vi "Winch.vi"() -> ()   [LabVIEW 2013]
uses:
  Globals/Homes.vi
  <vilib>/Rock Robotics/WPI/Joystick/WPI_JoystickGetSetRefNum.vi
  Robot Global Data.vi
  <vilib>/addons/control/pid/pid.llb/PID (DBL).vi
  <vilib>/addons/control/pid/NI_PID_pid.lvlib
panel:
  out "x-y":dbl
  out "Setpoint":dbl
  out "Motor Output":dbl
  out "Winch Voltage":dbl=2.9095941520000004
  in  "PID gains":T1={"proportional gain (Kc)"=2.75, "integral time (Ti, min)"=0.0, "derivative time (Td, min)"=0.0} {"derivative time (Td, min)" format="%.3f"; "integral time (Ti, min)" format="%.3f"; "proportional gain (Kc)" format="%.3f"}
  # "4.3"
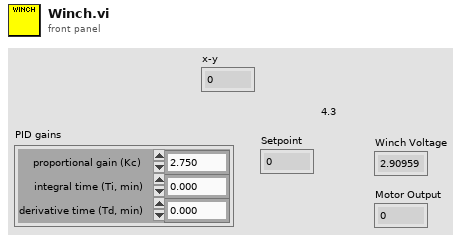
[diagram p1: front panel]
types:
  T1 = cluster{"proportional gain (Kc)":dbl, "integral time (Ti, min)":dbl, "derivative time (Td, min)":dbl}
  T2 = typedef "WPI_JoystickDevRef.ctl" = cluster{"Device":T3}
  T3 = typedef "WPI_JoystickDeviceEnum.ctl" = enum16{"USB 1", "USB 2", "USB 3", "USB 4", "Kinect 1", "Kinect 2"}
  T4 = typedef "WPI_AnalogChannelDevRef.ctl" = cluster{"DevStatus":errorcluster, "Analog Module":T5, "Analog Channel":T6}
  T5 = typedef "FPGA_TypedefAnalogModule.ctl" = enum16{"Analog Module 1", "Analog Module 2"}
  T6 = typedef "FPGA_AIChannel.ctl" = enum8{"AI 1", "AI 2", "AI 3", "AI 4", "AI 5", "AI 6", "AI 7", "AI 8", "Invalid"}
  T7 = typedef "WPI_MotorControlDeviceRef.ctl" = cluster{"DeviceStatus":errorcluster, "Type":enum16{"PWM", "CAN"}, "PWM":cluster{"Digital Module":T8, "PWM Channel":T9, "DeadBand":T10}, "CAN":cluster{"Device Number":u8, "Control Mode":T11, "Semaphore":T12, "Max Vout":dbl}, "Invert":bool, "TransformRef":T13, "InvTransformRef":T13}
  T8 = typedef "FPGA_TypedefDigitalModule.ctl" = enum16{"Digital Module 1", "Digital Module 2"}
  T9 = typedef "FPGA_DIOPWMChannel.ctl" = enum8{"PWM 1", "PWM 2", "PWM 3", "PWM 4", "PWM 5", "PWM 6", "PWM 7", "PWM 8", "PWM 9", "PWM 10", "Invalid"}
  T10 = typedef "WPI_PWMDeadband.ctl" = cluster{"Name":string, "maxPositivePwm":i32, "minPositivePwm":i32, "centerPwm":i32, "maxNegativePwm":i32, "minNegativePwm":i32, "angularRange":u16}
  T11 = typedef "WPI_CANJaguar_ControlMode.ctl" = enum8{"Percent VBus", "Current", "Speed", "Position", "Voltage"}
  T12 = typedef "Semaphore RefNum" = refnum<k1>
  T13 = typedef "WPI_PWMTransform_ConPane.ctl" = refnum<vi>
  T14 = typedef "WPI_DriverStationRobotMode2.ctl" = enum16{"Autonomous Disabled", "Autonomous Enabled", "Teleop Disabled", "Teleop Enabled", "Timeout", "Finish", "Test Disabled", "Test Enabled"}
  T15 = typedef "WPI_JoystickButtonState.ctl" = cluster{"Button 1":bool, "Button 2":bool, "Button 3":bool, "Button 4":bool, "Button 5":bool, "Button 6":bool, "Button 7":bool, "Button 8":bool, "Button 9":bool, "Button 10":bool, "Button 11":bool, "Button 12":bool}
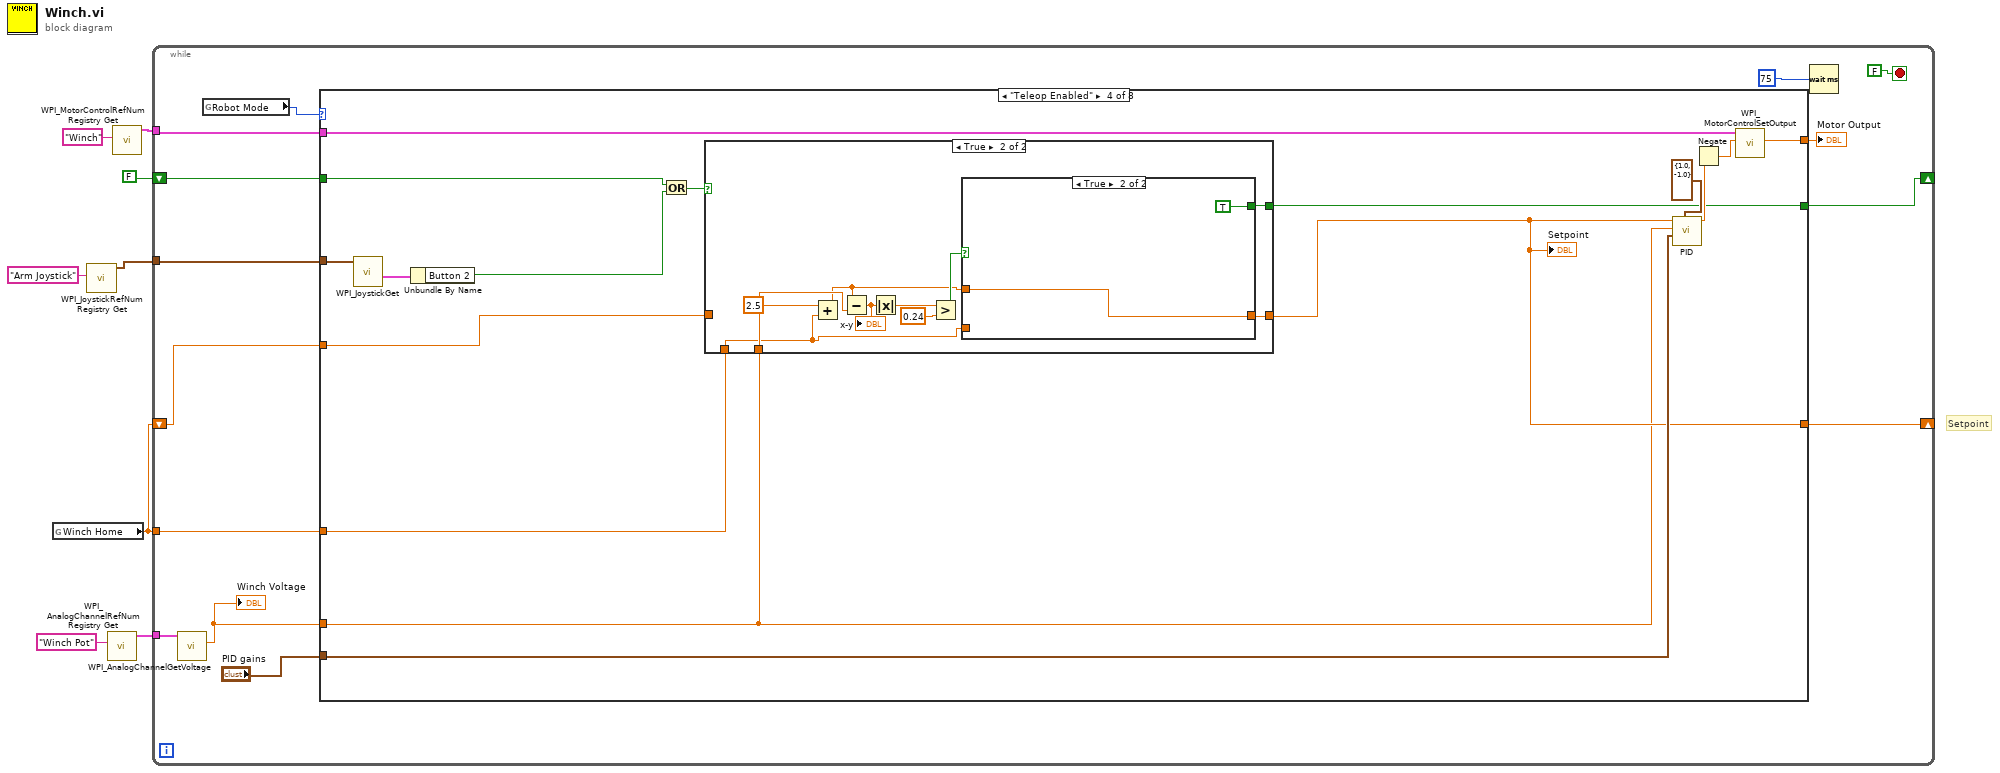
[diagram p0: block diagram]
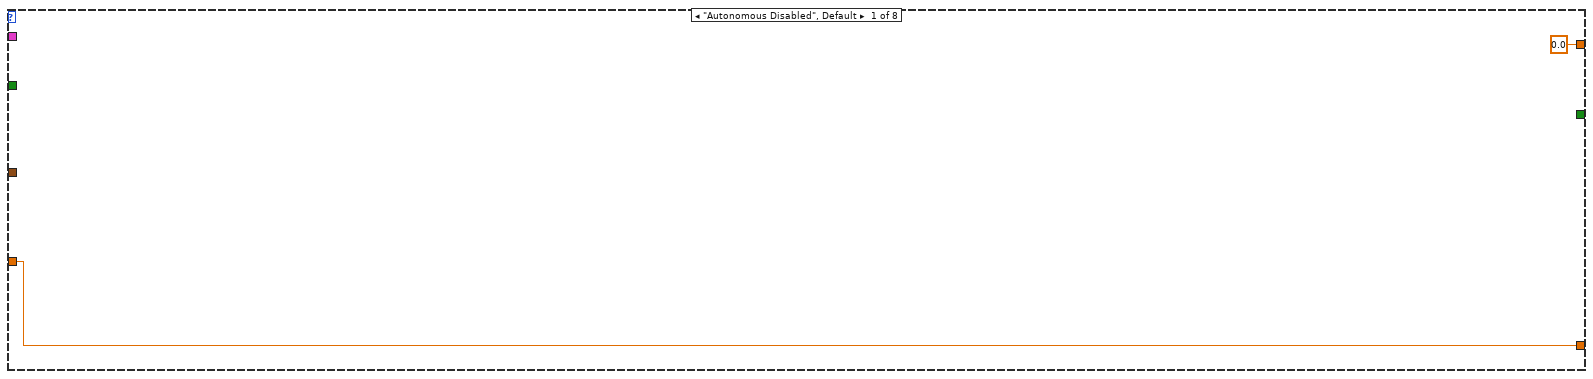
[diagram p2: hidden frame]
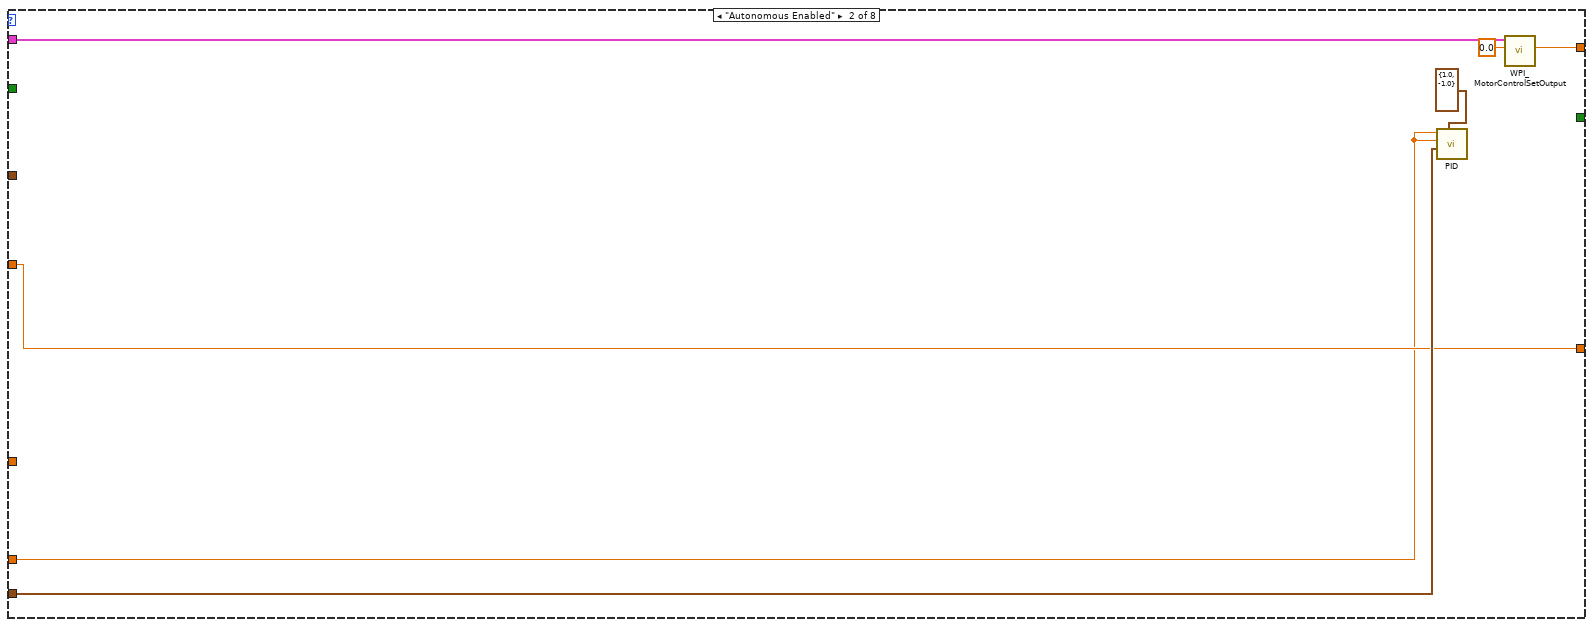
[diagram p3: hidden frame]
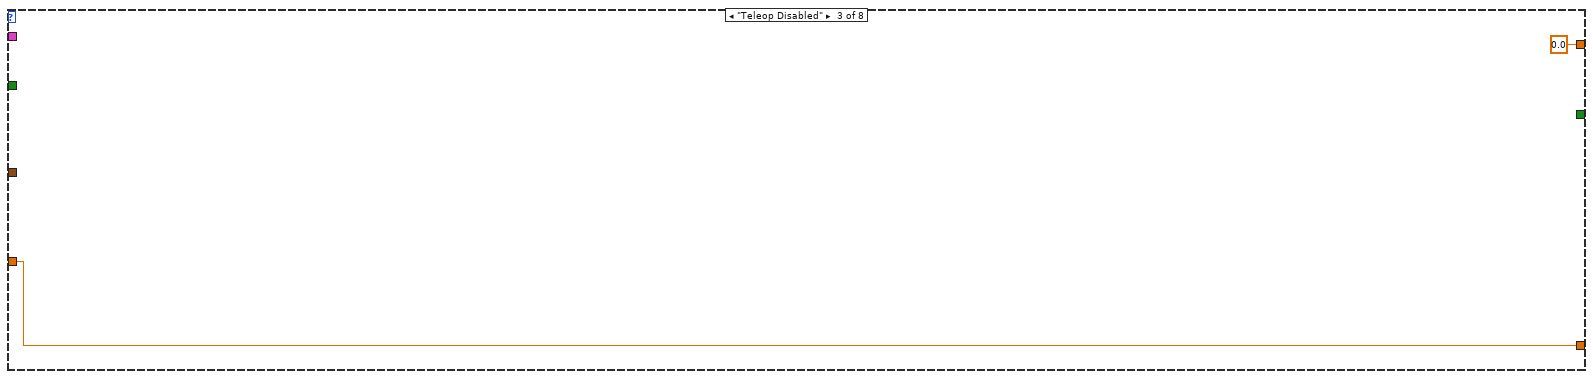
[diagram p4: hidden frame]
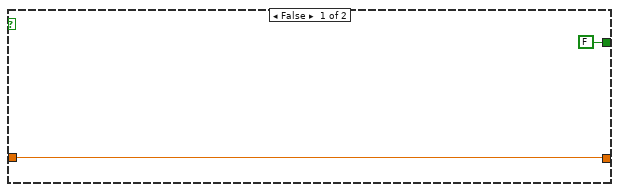
[diagram p5: hidden frame]
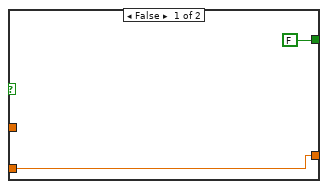
[diagram p6: hidden frame]
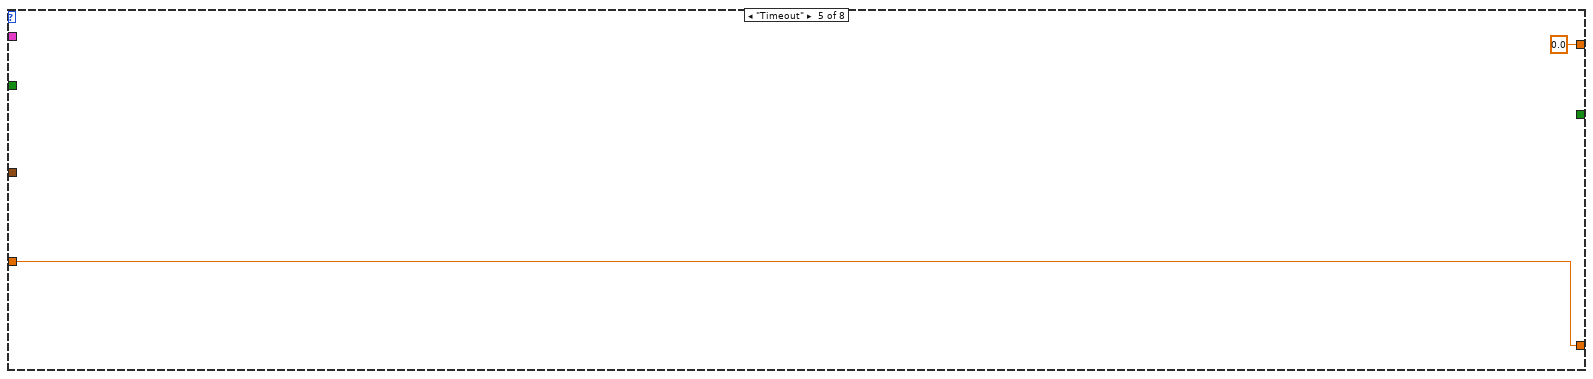
[diagram p7: hidden frame]
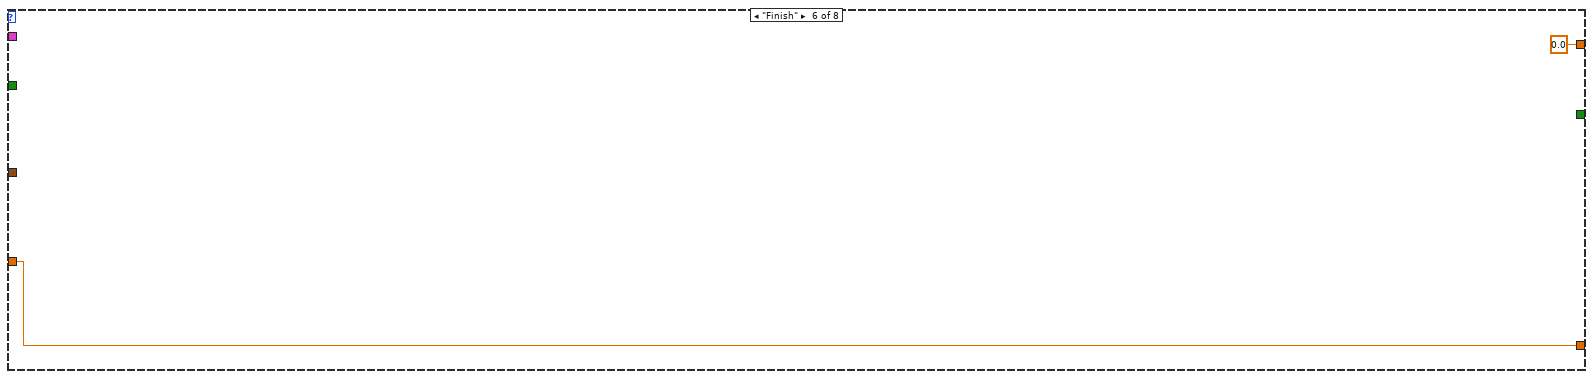
[diagram p8: hidden frame]
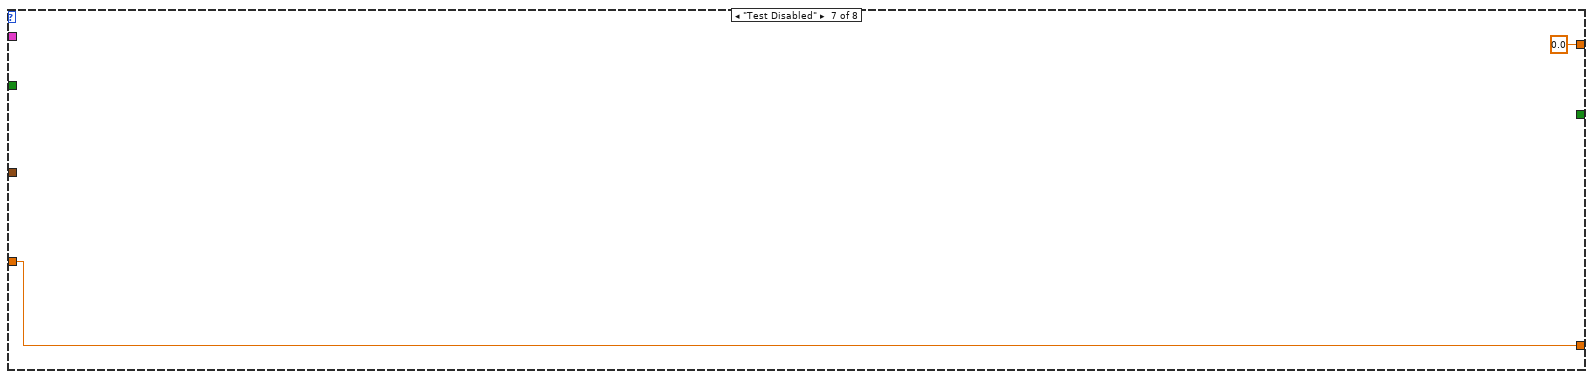
[diagram p9: hidden frame]
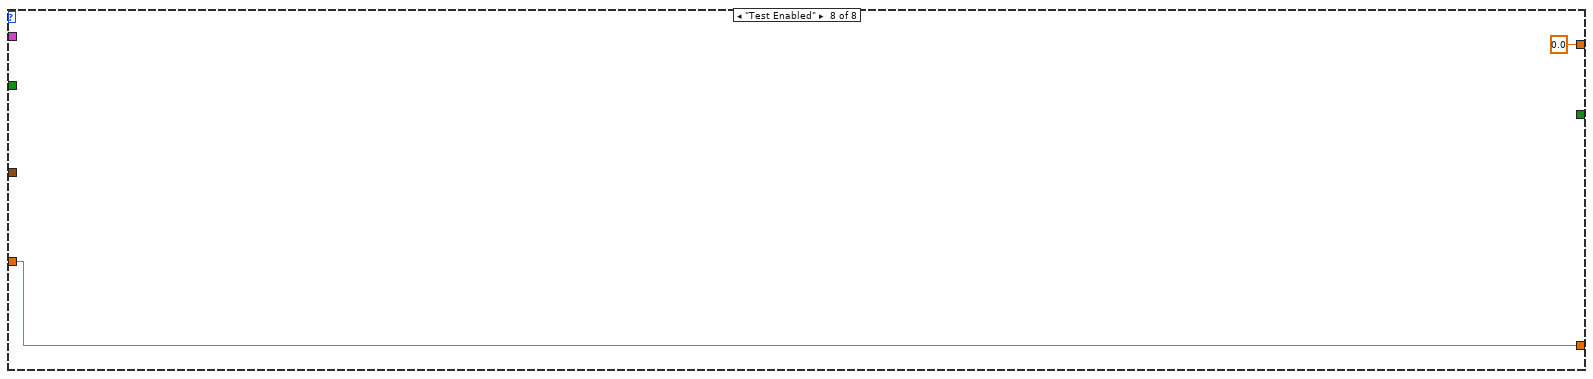
[diagram p10: hidden frame]
diagram:
  # "Setpoint"
  n1 = global read "Homes.vi" "Winch Home"() -> (w4:dbl)
  n2 = call <vilib>:"WPI_JoystickRefNum Registry Get.vi"("refnum name"="Arm Joystick") -> ("JoystickDevRef"=w2:T2)  [unwired: 9 in, 1 out]
  n3 = call <vilib>:"WPI_AnalogChannelRefNum Registry Get.vi"("refnum name"="Winch Pot") -> ("AIDeviceRef"=w8:T4)  [unwired: 9 in, 1 out]
  n4 = call <vilib>:"WPI_MotorControlRefNum Registry Get.vi"("refnum name"="Winch") -> ("MotorControlDevRef"=w5:T7)  [unwired: 9 in, 1 out]
  n5 = while {
    tunnel: w8 -> [w20]
    tunnel: w5 -> [w18]
    tunnel: w4 -> [w12]
    shift-right: [w11] -> _
    shift-left: w4 -> [w13]
    tunnel: w2 -> [w14]
    shift-right: [w9] -> _
    shift-left: FALSE ("Button 2") -> [w10]
    stop <- FALSE stop-if-true
    n6 = call <vilib>:"WPI_AnalogChannelGetVoltage.vi"("AIDeviceRef"=w20) -> ("Voltage"=w17:dbl)  [unwired: 8 in, 2 out]
    "Winch Voltage" <- w17
    n7 = global read "Robot Global Data.vi" "Robot Mode"() -> (w19:T14)
    n8 = case shown="\"Teleop Enabled\"" w19 {
      tunnel: w18 -> [_ w29 _ w48 _ _ _ _]
      tunnel: w17 -> [_ w26 _ w36 _ _ _ _]
      tunnel: "PID gains" -> [_ w30 _ w47 _ _ _ _]
      tunnel: [0.0 ("Motor Output") w28 0.0 ("Motor Output") w46 0.0 ("Motor Output") 0.0 ("Motor Output") 0.0 ("Motor Output") 0.0 ("Motor Output")] -> w15
      tunnel: w14 -> [_ _ _ w44 _ _ _ _]
      tunnel: w13 -> [w23 w27 w32 w40 w66 w68 w70 w72]
      tunnel: w12 -> [_ _ _ w42 _ _ _ _]
      tunnel: [w23 w27 w32 w41 w66 w68 w70 w72] -> w11
      tunnel: w10 -> [_ _ _ w37 _ _ _ _]
      tunnel: [_ _ _ w35 _ _ _ _] -> w9
      frame "Autonomous Disabled", Default {
      }
      frame "Autonomous Enabled" {
        n9 = call-poly <vilib>:"PID.vi"("output range"=cluster{"output high":dbl, "output low":dbl} {"output high"=1.0, "output low"=-1.0}, "PID gains"=w30, "process variable"=w26, "setpoint"=w26) -> ()  [unwired: 6 in, 2 out]
        n10 = call <vilib>:"WPI_MotorControlSetOutput.vi"("Output"=0.0, "MotorControlDevRef"=w29) -> ("Motor Output"=w28:dbl)  [unwired: 7 in, 2 out]
      }
      frame "Teleop Disabled" {
      }
      frame "Teleop Enabled" {
        n11 = call <vilib>:"WPI_JoystickGet.vi"("JoystickDevRef"=w44) -> ("Buttons"=w43:T15)  [unwired: 4 in, 2 out]
        n12 = Unbundle By Name(w43) -> ("Button 2"=w38:bool)
        n13 = Or(x=w37, y=w38) -> (x .or. y?=w39:bool)
        n14 = case shown="True" w39 {
          tunnel: w42 -> [_ w53]
          tunnel: [w51 w55] -> w41
          tunnel: w40 -> [w51 _]
          tunnel: w36 -> [_ w60]
          tunnel: [FALSE w52] -> w35
          frame False {
          }
          frame True {
            n15 = Add(x=2.5 ("Offset"), y=w53) -> (x+y=w54:dbl)
            n16 = Subtract(x=w54, y=w60) -> (x-y=w59:dbl)
            "x-y" <- w59
            n17 = Absolute Value(x=w59) -> (abs(x)=w58:dbl)
            n18 = Greater?(x=w58, y=0.24) -> (0:w56:bool)
            n19 = case shown="True" w56 {
              tunnel: [w63 w65] -> w55
              tunnel: w54 -> [_ w65]
              tunnel: w53 -> [w63 _]
              tunnel: [FALSE TRUE] -> w52
              frame False {
              }
              frame True {
              }
            }
          }
        }
        "Setpoint" <- w41
        n20 = call-poly <vilib>:"PID.vi"("output range"=cluster{"output high":dbl, "output low":dbl} {"output high"=1.0, "output low"=-1.0}, "PID gains"=w47, "process variable"=w36, "setpoint"=w41) -> ("output"=w45:dbl)  [unwired: 6 in, 1 out]
        n21 = Negate(x=w45) -> (-x=w34:dbl)
        n22 = call <vilib>:"WPI_MotorControlSetOutput.vi"("Output"=w34, "MotorControlDevRef"=w48) -> ("Motor Output"=w46:dbl)  [unwired: 7 in, 2 out]
      }
      frame "Timeout" {
      }
      frame "Finish" {
      }
      frame "Test Disabled" {
      }
      frame "Test Enabled" {
      }
    }
    "Motor Output" <- w15
    n23 = Wait (ms)(milliseconds to wait=u32 75) -> ()  [unwired: 1 out]
  }
